vi "Write ShopAssistant's Enqueuer.vi"(8 "error in (no error)":errorcluster, 10 "Actor Framework:Message Enqueuer":refnum<class "Message Enqueuer.lvclass">, 11 "Customer A in":refnum<class "Customer A.lvclass">) -> (0 "error out":errorcluster, 3 "Customer A out":refnum<class "Customer A.lvclass">)   [LabVIEW 2020, in "Customer A.lvlib" / "Customer A.lvclass"]
uses:
  Customer A.lvclass
  <vilib>/ActorFramework/Message Enqueuer/Message Enqueuer.lvclass
  Customer A.lvclass/Customer A.ctl
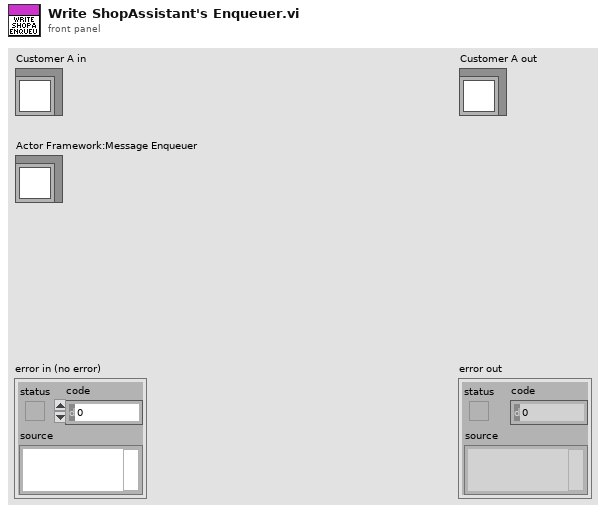
[diagram p1: front panel]
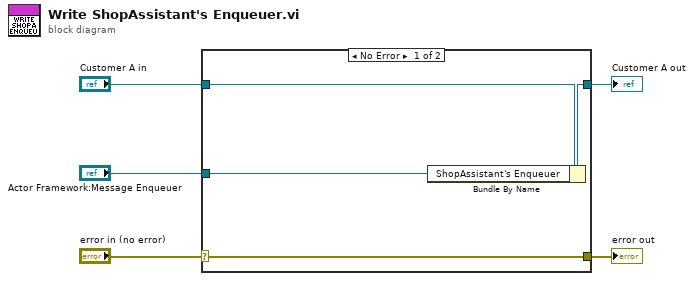
[diagram p0: block diagram]
diagram:
  n1 = case shown="No Error" "error in (no error)" {
    selector: "error in (no error)" -> [w9 w10]
    tunnel: [w9 w10] -> w4
    tunnel: [w7 w11] -> w2
    tunnel: "Customer A in" -> [w8 w11]
    tunnel: "Actor Framework:Message Enqueuer" -> [w6 _]
    frame No Error {
      n2 = Bundle By Name(cluster=w8, "ShopAssistant's Enqueuer"=w6) -> (w7:refnum<class "Customer A.lvclass">)
    }
    frame Error {
    }
  }
  "error out" <- w4
  "Customer A out" <- w2
